vi "Get All Keys.vi"(8 "error in (no error)":errorcluster, 11 "Configuration File In":refnum<class "Configuration File.lvclass">) -> (0 "error out":errorcluster, 1 "Keys":string[](array[string]), 3 "Configuration File Out":refnum<class "Configuration File.lvclass">)   [LabVIEW 2020, in "Configuration File.lvclass"]
doc: "High-level function for reading configuration file data from process class."
uses:
  Configuration File.lvclass
  <vilib>/Utility/config.llb/NI_LVConfig.lvlib
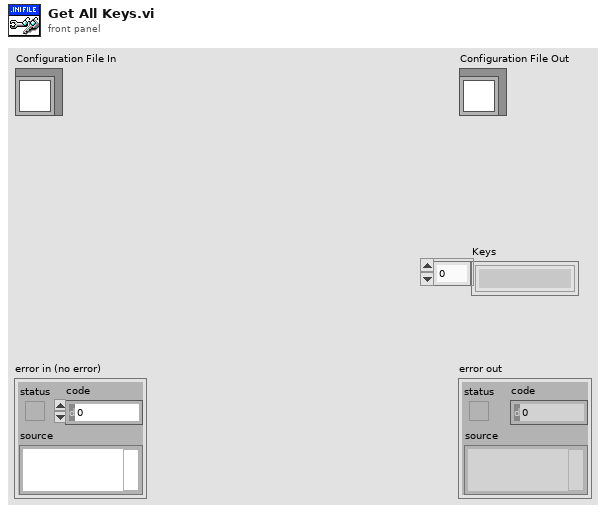
[diagram p1: front panel]
types:
  T1 = typedef "NI_LVConfig.lvlib/Config Data RefNum.ctl" = refnum<k1>
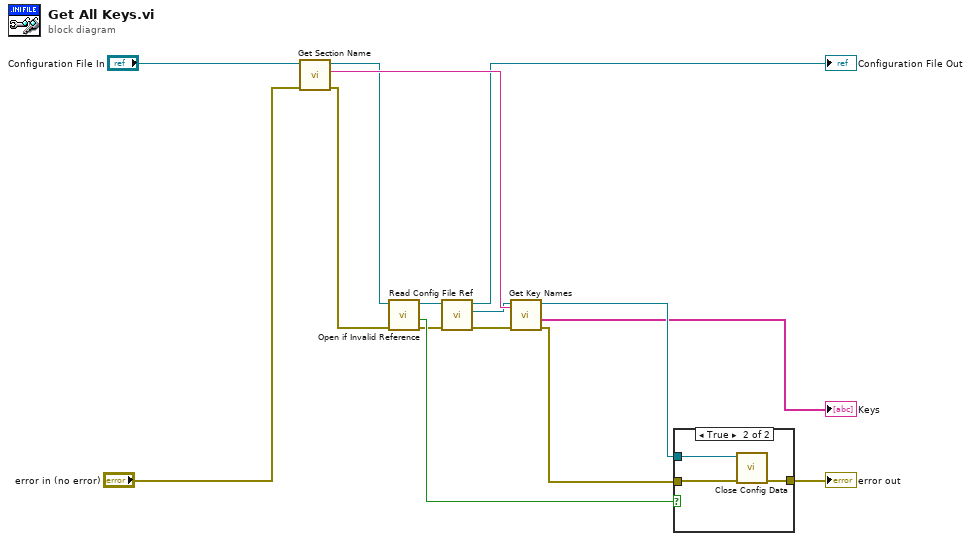
[diagram p0: block diagram]
diagram:
  n1 = call "Get Section Name.vi"("error in (no error)"="error in (no error)", "Configuration File In"="Configuration File In") -> ("error out"=w8:errorcluster, "Section Name"=w11:string, "Configuration File Out"=w10:refnum<class "Configuration File.lvclass">)  [unwired: 7 in]
  n2 = call "Open if Invalid Reference.vi"("error in (no error)"=w8, "Configuration File In"=w10) -> ("error out"=w3:errorcluster, "File opened?"=w6:bool, "Configuration File Out"=w9:refnum<class "Configuration File.lvclass">)  [unwired: 6 in, 1 out]
  n3 = call "Read Config File Ref.vi"("error in (no error)"=w3, "Configuration File In"=w9) -> ("error out"=w2:errorcluster, "refnum out"=w1:T1, "Configuration File Out"=→"Configuration File Out":refnum<class "Configuration File.lvclass">)  [unwired: 7 in]
  n4 = call <vilib>:"Get Key Names.vi"("section"=w11, "error in (no error)"=w2, "refnum"=w1) -> ("error out"=w12:errorcluster, "key names"=→"Keys":string[], "refnum out"=w13:T1)  [unwired: 5 in, 1 out]
  n5 = case shown="True" w6 {
    tunnel: w13 -> [_ w19]
    tunnel: w12 -> [w16 w18]
    tunnel: [w16 w17] -> w7
    frame False {
    }
    frame True {
      n6 = call <vilib>:"Close Config Data.vi"("error in (no error)"=w18, "refnum"=w19) -> ("error out"=w17:errorcluster)  [unwired: 8 in, 1 out]
    }
  }
  "error out" <- w7
